vi "Set Voltage.vi"(8 "error in (no error)":errorcluster, 10 "Voltage":dbl, 11 "Analog-Output in":refnum<class "Analog-Output.lvclass">) -> (0 "error out":errorcluster, 3 "Analog-Output out":refnum<class "Analog-Output.lvclass">)   [LabVIEW 2019, in "Analog-Output.lvlib" / "Analog-Output.lvclass"]
uses:
  Library/Analog-Output.lvclass
  C:/Users/Public/Documents/Development/builds/Engine/Monitored Actor.lvlibp/Monitored Actor/Monitored Actor/Monitored Actor.lvclass
  C:/Users/Public/Documents/Development/builds/Instruments/Instruments.lvlibp/Library/Instruments.lvclass
  Library/Analog-Output.lvclass/Analog-Output.ctl
  Read Settings_All.vi
  Read Measured Table.vi
  Write Settings_All.vi
  Read Limit.vi
  builds/Engine/Monitored Actor.lvlibp/Monitored Actor/Monitored Actor/Read Actor Label.vi
  builds/Instruments/Instruments.lvlibp/Private/Polymorphic/Integers/Event from DBL.vi
  builds/Instruments/Instruments.lvlibp/Accessors/Command with Logging.vi
  builds/Instruments/Instruments.lvlibp/Library/Instruments.lvclass
  builds/Instruments/Instruments.lvlibp
  builds/Engine/Engine.lvlibp/Project/Engine.lvclass
  C:/Users/Public/Documents/Development/builds/Engine/Engine.lvlibp/Project/Engine.lvclass
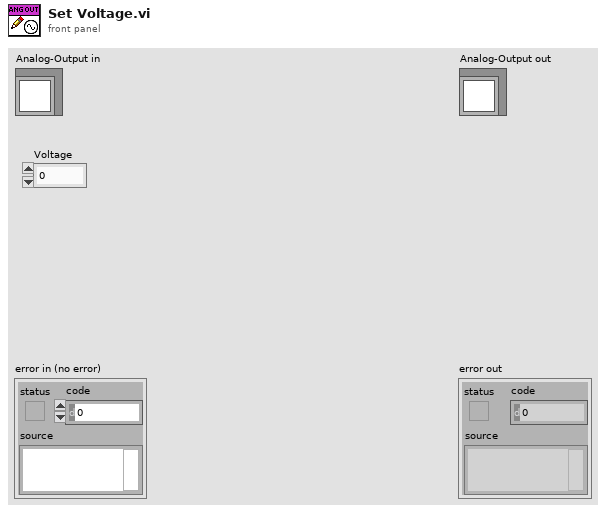
[diagram p1: front panel]
types:
  T1 = typedef "Analog-Output.lvlib/Analog-Output.lvclass/Settings.ctl" = cluster{"Voltage":dbl}
  T2 = cluster{"Timestamp":timestamp, "Description":string, "Data":string}
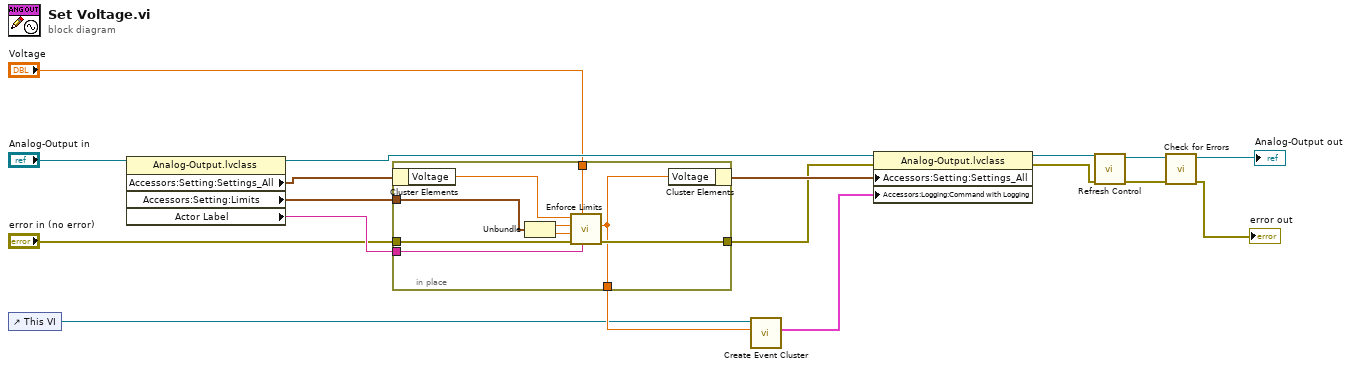
[diagram p0: block diagram]
diagram:
  n1 = control-ref of="This VI"() -> (w13:refnum<vi>)
  n2 = property class="Analog-Output.lvclass"(reference="Analog-Output in") -> (reference out=w12:refnum<class "Analog-Output.lvclass">, "Accessors:Setting:Settings_All"=w16:T1, "Accessors:Setting:Limits"=w5:cluster{"Max_V":dbl, "Min_V":dbl}, "Actor Label"=w15:string)  [unwired: 1 in, 1 out]
  n3 = in-place {
    in-place-border: [w27] -> w1
    in-place-border: w15 -> [w26]
    in-place-border: "error in (no error)" -> [w25]
    in-place-border: [w24] -> w18
    in-place-border: w5 -> [w23]
    in-place-border: "Voltage" -> [w19]
    n4 = in-place-cluster #1(w16) -> ("Voltage"=w20:dbl)
    n5 = Unbundle(w23) -> ("Max_V"=w22:dbl, "Min_V"=w21:dbl)
    n6 = call "Enforce Limits.vi"("Device"=w26, "Setpoint"=w19, "error in"=w25, "Minimum"=w21, "Maximum"=w22, "Previous"=w20) -> ("error out"=w27:errorcluster, "Protected Setpoint"=w24:dbl)  [unwired: 4 in]
    n7 = in-place-cluster #1("Voltage"=w24) -> (w6:T1)
  }
  n8 = call-poly "Create Event Cluster.vi"("Value"=w18, "VI Refnum"=w13) -> ("Event Data"=w7:T2)  [unwired: 9 in]
  n9 = property class="Analog-Output.lvclass"(reference=w12, error in=w1, "Accessors:Setting:Settings_All"=w6, "Accessors:Logging:Command with Logging"=w7) -> (reference out=w2:refnum<class "Analog-Output.lvclass">, error out=w8:errorcluster)
  n10 = call "Refresh Control.vi"("error in (no error)"=w8, "Analog-Output in"=w2) -> ("error out"=w9:errorcluster, "Analog-Output out"=w11:refnum<class "Analog-Output.lvclass">)  [unwired: 8 in]
  n11 = call "Check for Errors.vi"("error in"=w9, "Engine in"=w11) -> ("error out"=→"error out":errorcluster, "Engine out"=→"Analog-Output out":refnum<class "Analog-Output.lvclass">)  [unwired: 8 in]
